vi "Action.vi"(7 "Assert Message":T1, 8 "error in (no error)":errorcluster, 11 "Log To File in":refnum<class "Log To File.lvclass">) -> (0 "error out":errorcluster)   [LabVIEW 2018, in "Assert API Components.lvlib" / "Log Assert Core.lvlib" / "Log To File.lvclass"]
doc: "Dynamic dispatch vi which is triggered when an assert fails and the failure action is set to Log to File.\nLogs the Assert failure details to file and moves on."
uses:
  Log To File.lvclass
  Message Data.ctl
  Failure Actions.ctl
  <vilib>/Utility/sysdir.llb/System Directory Type.ctl
  <vilib>/Utility/file.llb/Write Delimited Spreadsheet (string).vi
  Assert API Components.lvlib
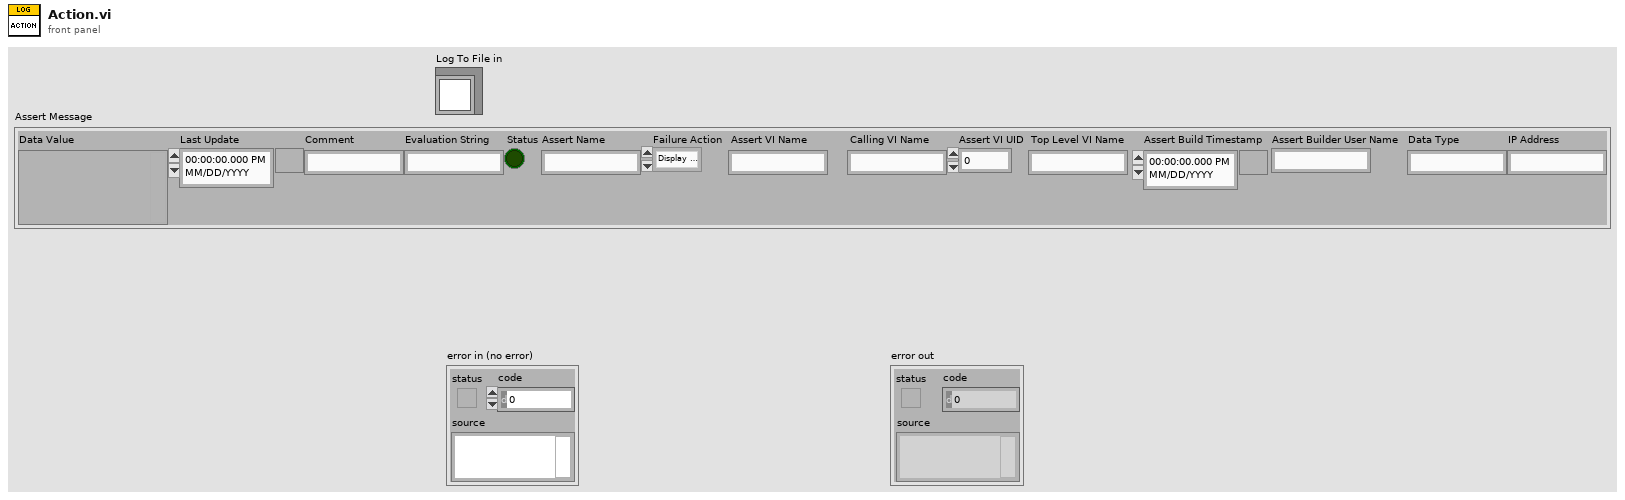
[diagram p1: front panel]
types:
  T1 = typedef "Assert API Components.lvlib/Message Data.ctl" = cluster{"Data Value":variant, "Last Update":timestamp, "Comment":string, "Evaluation String":string, "Status":bool, "Assert Name":string, "Failure Action":T2, "Assert VI Name":string, "Calling VI Name":string, "Assert VI UID":i32, "Top Level VI Name":string, "Assert Build Timestamp":timestamp, "Assert Builder User Name":string, "Data Type":string, "IP Address":string}
  T2 = typedef "Assert API Components.lvlib/Failure Actions.ctl" = enum16{"Display Only", "Log To File", "Pause Execution", "Abort Execution"}
  T3 = typedef "System Directory Type.ctl" = i32
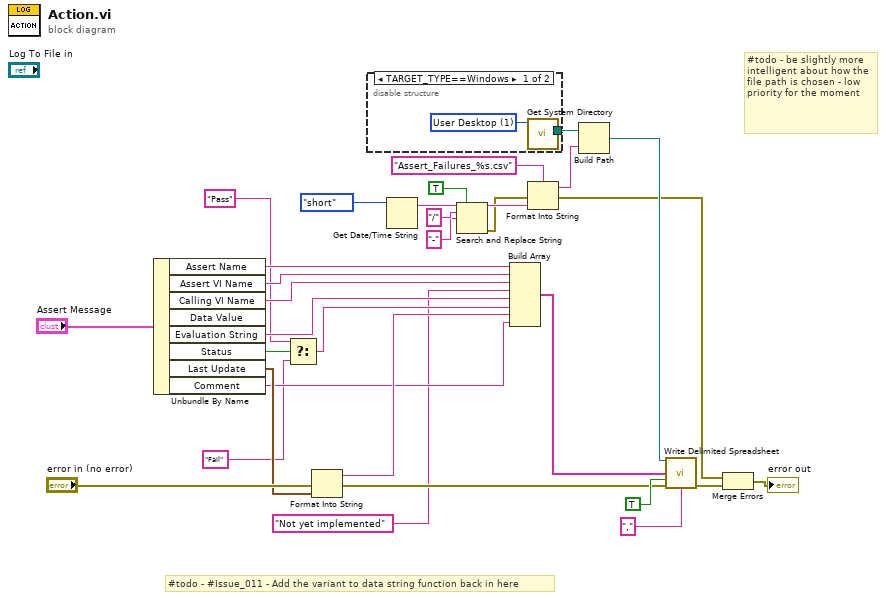
[diagram p0: block diagram]
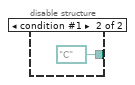
[diagram p2: hidden frame]
diagram:
  # "#todo - #Issue_011 - Add the variant to data string function back in here"
  # "#todo - be slightly more intelligent about how the file path is chosen - low priority for the moment"
  n1 = Unbundle By Name("Assert Message") -> ("Assert Name"=w12:string, "Assert VI Name"=w11:string, "Calling VI Name"=w10:string, "Evaluation String"=w9:string, "Status"=w5:bool, "Last Update"=w13:timestamp, "Comment"=w7:string)  [unwired: 1 out]
  n2 = Select(t="Pass", s=w5, f="Fail") -> (s? t:f=w2:string)
  n3 = Format Into String(error in="error in (no error)", w13) -> (resulting string=w8:string, error out=w14:errorcluster)  [unwired: 2 in]
  n4 = disable-structure shown="TARGET_TYPE==Windows" {
    disable-tunnel: [w33 path "C:/" ("system directory")] -> w23
    frame condition #0 (active) {
      w34 = T3 1 items=["User Home"=0, "User Desktop"=1, "User Documents"=2, "User Application Data"=3, "User Preferences"=4, "User Temporary"=5, "Public Documents"=6, "Public Application Data"=7, "Public Preferences"=8, "Public Cache"=13, "System Core Libraries"=9, "System Installed Libraries"=10, "Application Files"=11, "Boot Volume Root"=12] ("system directory type")
      n5 = call <vilib>:"Get System Directory.vi"("system directory type"=w34) -> ("system directory"=w33:path)  [unwired: 10 in]
    }
    frame condition #1 {
    }
  }
  n6 = Get Date/Time String(date format (0)=enum16{"short", "long", "abbreviated"}."short") -> (date string=w29:string)  [unwired: 2 in, 1 out]
  n7 = Search and Replace String(replace all?=TRUE ("replace all? (F)"), input string=w29, search string="/", replace string="-" ("replace string (\"\")")) -> (result string=w26:string, error out=w19:errorcluster)  [unwired: 4 in, 2 out]
  n8 = Build Array(w12, w11, w10, "Not yet implemented" ("element"), w9, w2, w8, w7) -> (w6:string[])
  n9 = Format Into String(format string="Assert_Failures_%s.csv", error in=w19, w26) -> (resulting string=w24:string, error out=w17:errorcluster)  [unwired: 1 in]
  n10 = Build Path(base path=w23, name or relative path=w24) -> (appended path=w22:path)
  n11 = call-poly <vilib>:"Write Delimited Spreadsheet.vi"("file path (dialog if empty)"=w22, "1D data"=w6, "append to file? (new file:F)"=TRUE, "error in (no error)"=w14, "delimiter (\\t)"="," ("delimiter (\\t)")) -> ("error out"=w30:errorcluster)  [unwired: 9 in, 1 out]
  n12 = Merge Errors(w17, w30) -> (→"error out":errorcluster)
